vi "Get Matrix - file.vi"(7 "is string?":bool, 8 "error in (no error)":errorcluster, 10 "variable name":string, 11 "GOLPI ref. in":T1={"pipe handle"={"lv_proc.dll file path"=path "", "process instance handle"=[], "debug mode"=FALSE, "debug data"=[]}, "fast read timeout [ms]"=500, "fast read settle time [ms]"=10, "fast read to multiple [ms]"=1, "max elements per input line"=100, "slow read timeout [ms]"=5000, "stdin double format specifier"="%_16e", "max elements per stdout output column"=100, "console mode bitstream"=FALSE, "bitstream first read timeout [ms]"=1000, "bitstream read timeout [ms]"=50, "struct transfer possible"=FALSE, "matlab mode"=FALSE}) -> (0 "error out":errorcluster, 1 "cmplx double array":cdb[][](array[numeric]), 2 "double array":dbl[][](array[numeric]), 3 "GOLPI ref. out":T1={"pipe handle"={"lv_proc.dll file path"=path "", "process instance handle"=[], "debug mode"=FALSE, "debug data"=[]}, "fast read timeout [ms]"=500, "fast read settle time [ms]"=10, "fast read to multiple [ms]"=1, "max elements per input line"=100, "slow read timeout [ms]"=5000, "stdin double format specifier"="%_16e", "max elements per stdout output column"=100, "console mode bitstream"=FALSE, "bitstream first read timeout [ms]"=1000, "bitstream read timeout [ms]"=50, "struct transfer possible"=FALSE, "matlab mode"=FALSE}, 5 "string array":string[](array[string]))   [LabVIEW 2020, in "GOLPI library.lvlib"]
doc: "Saves GNU Octave variable into temporary file and loads it into LabVIEW. The variable is at the output terminal according to type of variable. Supported are reals (doubles), complex and strings. One has to select whether the variable is string."
uses:
  GOLPI library.lvlib
  GOLPI reference Type Def.ctl
  Pipe Handle.ctl
  Custom Error Codes Enum Type Def.vi
  LV Process library.lvlib
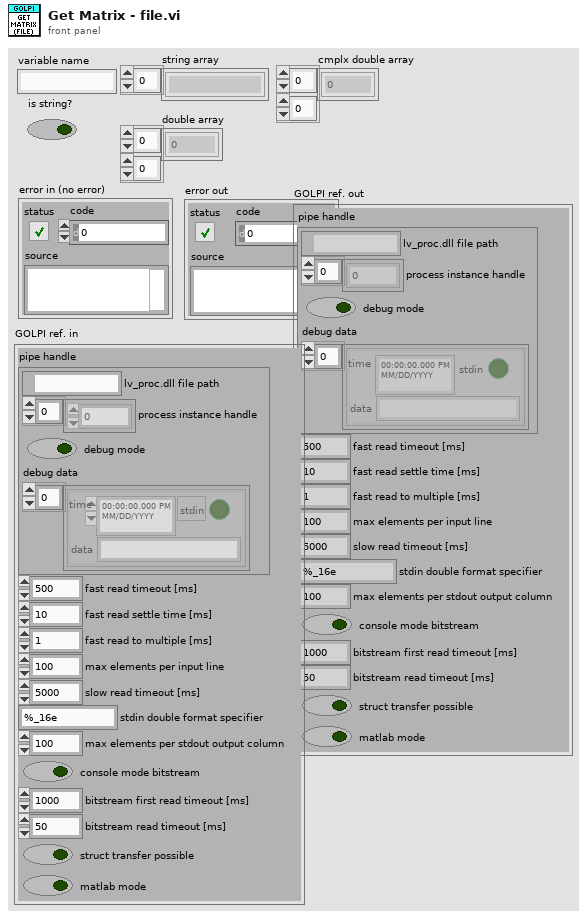
[diagram p1: front panel]
types:
  T1 = typedef "GOLPI library.lvlib/GOLPI reference Type Def.ctl" = cluster{"pipe handle":T2, "fast read timeout [ms]":u32, "fast read settle time [ms]":u32, "fast read to multiple [ms]":u32, "max elements per input line":u32, "slow read timeout [ms]":u32, "stdin double format specifier":string, "max elements per stdout output column":u32, "console mode bitstream":bool, "bitstream first read timeout [ms]":u32, "bitstream read timeout [ms]":u32, "struct transfer possible":bool, "matlab mode":bool}
  T2 = typedef "LV Process library.lvlib/Pipe Handle.ctl" = cluster{"lv_proc.dll file path":path, "process instance handle":u32[], "debug mode":bool, "debug data":cluster{"time":timestamp, "stdin":bool, "data":string}[]}
  T3 = typedef "GOLPI library.lvlib/Custom Error Codes Enum Type Def.vi" = enum16{"no error", "00 working directory PAR1 missing", "01 octave binary PAR1 missing", "02 octave report error PAR1", "03 empty output last cmd PAR1", "04 missing temporary file PAR1", "05 pwd PAR 1 not exist", "06 oct package not installed", "07 octave default binary missing", "10 var PAR1 not string, vect", "11 var PAR1 not num, scal, ~compl", "12 var PAR1 not num, scal, compl", "13 var PAR1 not num, vect, ~compl", "14 var PAR1 not num, vect, compl", "15 var PAR1 not num, mat, ~compl", "16 var PAR1 not num, mat, ~compl", "30 read timeout", "60 bitstream transport failed", "61 bitstream decode error PAR1", "62 bitstream cannot be set", "70 struct transfer not possible", "80 struct: cluster elem. PAR1 not implem.", "81 struct: structure field PAR1 not implem.", "82 struct: size mismatch of PAR1", "83 struct: type mismatch of PAR1", "98 internal error", "99 not finished", "90 Not supported in Matlab mode", "91 Matlab variable transfer error", "92 Matlab Script Error"}
  T4 = enum16{"open", "replace", "create", "open or create", "replace or create", "replace or create with confirmation"}
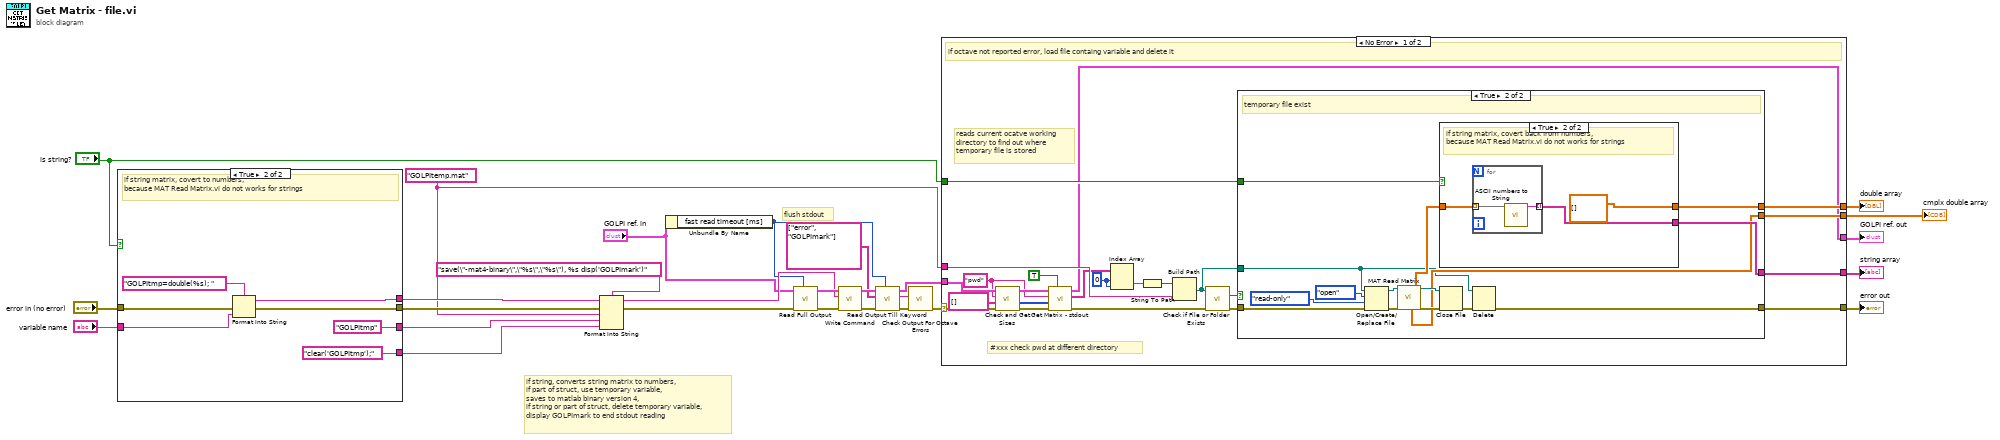
[diagram p0: block diagram]
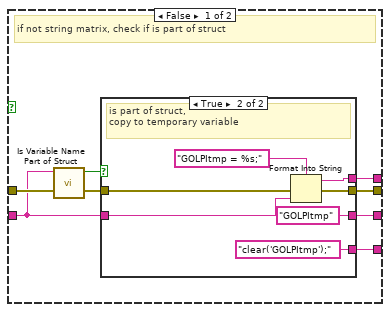
[diagram p2: hidden frame]
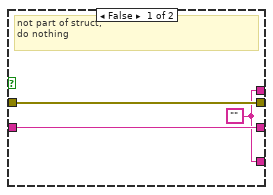
[diagram p3: hidden frame]
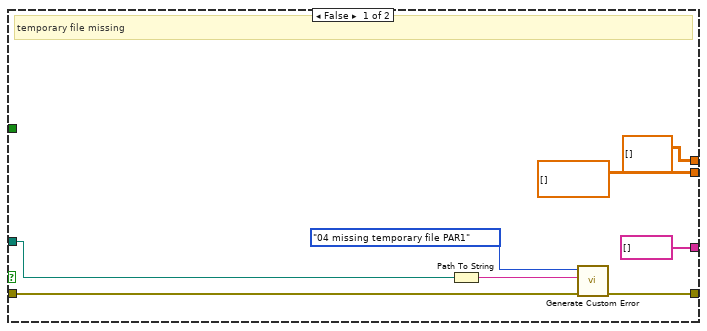
[diagram p4: hidden frame]
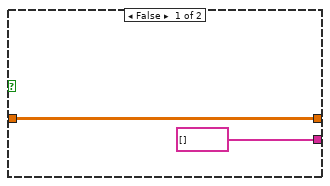
[diagram p5: hidden frame]
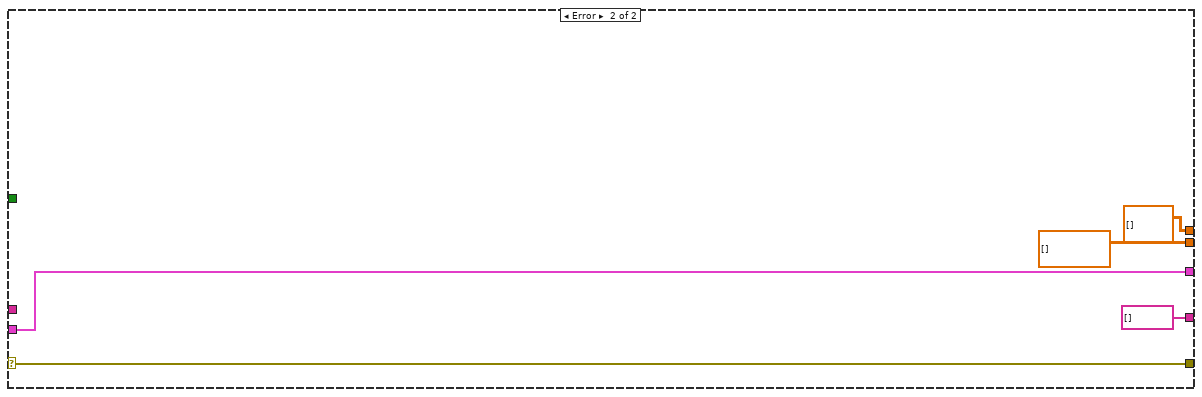
[diagram p6: hidden frame]
diagram:
  w7 = "GOLPItemp.mat" ("name or relative path")
  # "if string, converts string matrix to numbers,\nif part of struct, use temporary variable,\nsaves to matlab binary version 4,\nif string or part of struct, delete temporary variable,\ndisplay GOLPImark to end stdout reading"
  # "flush stdout"
  n1 = case shown="True" "is string?" {
    tunnel: [w33 w50] -> w14
    tunnel: [w30 "GOLPItmp" ("format string")] -> w15
    tunnel: "variable name" -> [w29 w48]
    tunnel: [w32 w46] -> w13
    tunnel: "error in (no error)" -> [w31 w47]
    tunnel: [w28 "clear('GOLPItmp');" ("format string")] -> w1
    frame False {
      # "if not string matrix, check if is part of struct"
      n2 = call "Is Variable Name Part of Struct.vi"("variable name"=w29) -> ("Is part of struct?"=w34:bool)  [unwired: 10 in]
      n3 = case shown="True" w34 {
        tunnel: [w35 w38] -> w33
        tunnel: [w37 w39] -> w32
        tunnel: w31 -> [w37 w40]
        tunnel: [w36 "GOLPItmp" ("f")] -> w30
        tunnel: w29 -> [w36 w41]
        tunnel: [w35 "clear('GOLPItmp');" ("format string")] -> w28
        frame False {
          w35 = ""
          # "not part of struct,\ndo nothing"
        }
        frame True {
          # "is part of struct,\ncopy to temporary variable"
          n4 = Format Into String(format string="GOLPItmp = %s;" ("f"), error in=w40, w41) -> (resulting string=w38:string, error out=w39:errorcluster)  [unwired: 1 in]
        }
      }
    }
    frame True {
      # "if string matrix, covert to numbers,\nbecause MAT Read Matrix.vi do not works for strings"
      n5 = Format Into String(format string="GOLPItmp=double(%s); ", error in=w47, w48) -> (resulting string=w50:string, error out=w46:errorcluster)  [unwired: 1 in]
    }
  }
  n6 = Format Into String(format string="save(\"-mat4-binary\",\"%s\",\"%s\"), %s disp('GOLPImark')", initial string=w14, error in=w13, w7, w15, w1) -> (resulting string=w18:string, error out=w24:errorcluster)
  n7 = Unbundle By Name("GOLPI ref. in") -> ("fast read timeout [ms]"=w4:u32)
  n8 = call "Read Full Output.vi"("timeout [ms]"=w4, "error in"=w24, "GOLPI ref. in"="GOLPI ref. in") -> ("error out"=w25:errorcluster, "GOLPI ref. out"=w26:T1)  [unwired: 5 in, 2 out]
  n9 = call "Write Command.vi"("error in"=w25, "command"=w18, "GOLPI ref. in"=w26) -> ("error out"=w23:errorcluster, "GOLPI ref. out"=w20:T1)  [unwired: 7 in]
  n10 = call "Read Output Till Keyword.vi"("timeout [ms]"=w4, "error in"=w23, "keywords"=string[] ["error", "GOLPImark"], "GOLPI ref. in"=w20) -> ("error out"=w22:errorcluster, "read buffer"=w21:string, "GOLPI ref. out"=w6:T1)  [unwired: 4 in, 1 out]
  n11 = call "Check Output For Octave Errors.vi"("error in"=w22, "read buffer"=w21) -> ("error out"=w17:errorcluster)  [unwired: 9 in]
  n12 = case shown="No Error" w17 {
    selector: w17 -> [w60 w109]
    tunnel: [w74 w109] -> w27
    tunnel: [w72 string[] []] -> w10
    tunnel: "is string?" -> [w73 _]
    tunnel: [w71 dbl[][] [] ("double array")] -> w9
    tunnel: [w70 cdb[][] [] ("CDB")] -> w8
    tunnel: w7 -> [w68 _]
    tunnel: w6 -> [w61 w105]
    tunnel: [w59 w105] -> w5
    frame No Error {
      w56 = 0 ("index (row)")
      w54 = "pwd" ("variable name")
      # "#xxx check pwd at different directory"
      # "reads current ocatve working\ndirectory to find out where\ntemporary file is stored"
      # "if octave not reported error, load file containg variable and delete it"
      n13 = call "Check and Get Sizes.vi"("error in (no error)"=w60, "test commands"=string[] [], "variable name"=w54, "GOLPI ref. in"=w61) -> ("error out"=w63:errorcluster, "octave sizes"=w53:i32[], "GOLPI ref. out"=w64:T1)  [unwired: 4 in, 1 out]
      n14 = call "Get Matrix - stdout.vi"("is string?"=TRUE ("is string"), "error in (no error)"=w63, "octave sizes"=w53, "variable name"=w54, "GOLPI ref. in"=w64) -> ("error out"=w58:errorcluster, "array"=w57:string[][], "GOLPI ref. out"=w59:T1)  [unwired: 4 in]
      n15 = Index Array(array=w57, index (row)=w56, index (col)=w56) -> (element=w55:string)
      n16 = String To Path(string=w55) -> (path=w69:path)
      n17 = Build Path(base path=w69, name or relative path=w68) -> (appended path=w66:path)
      n18 = call <vilib>:"Check if File or Folder Exists.vi"("error in (no error)"=w58, "path"=w66) -> ("error out"=w67:errorcluster, "file or folder exists?"=w65:bool)  [unwired: 7 in, 1 out]
      n19 = case shown="True" w65 {
        tunnel: [w81 w90] -> w74
        tunnel: w73 -> [_ w89]
        tunnel: [string[] [] w87] -> w72
        tunnel: [dbl[][] [] ("double array") w86] -> w71
        tunnel: [cdb[][] [] ("CDB") w85] -> w70
        tunnel: w67 -> [w82 w84]
        tunnel: w66 -> [w76 w83]
        frame False {
          # "temporary file missing"
          n20 = Path To String(path=w76) -> (string=w75:string)
          n21 = call "Generate Custom Error.vi"("error in"=w82, "PAR1"=w75, "GOLPI error"=Custom_Error_Codes_Enum_Type_Def.vi."04 missing temporary file PAR1" ("Enum")) -> ("error out"=w81:errorcluster)  [unwired: 8 in]
        }
        frame True {
          # "temporary file exist"
          n22 = Open/Create/Replace File(file path (use dialog)=w83, error in=w84, operation (0:open)=T4."open", access (0:read/write)=enum16{"read/write", "read-only", "write-only"}."read-only") -> (refnum out=w94:refnum<file>, error out=w96:errorcluster)  [unwired: 2 in, 1 out]
          n23 = call "MAT Read Matrix.vi"("Ref Num"=w94, "Error In"=w96) -> ("CDB"=w85:cdb[][], "DBL"=w88:dbl[][], "Dup Ref Num"=w95:refnum<file>, "error out"=w97:errorcluster)  [unwired: 5 in, 9 out]
          n24 = case shown="True" w89 {
            tunnel: w88 -> [w98 w102]
            tunnel: [string[] [] w101] -> w87
            tunnel: [w98 dbl[][] [] ("double array")] -> w86
            frame False {
            }
            frame True {
              # "if string matrix, covert back from numbers,\nbecause MAT Read Matrix.vi do not works for strings"
              n25 = for {
                tunnel: [w103] -> w101 mode=indexing
                tunnel: w102 -> [w104] mode=indexing
                n26 = call "ASCII numbers to String.vi"("ascii numbers"=w104) -> ("string"=w103:string)  [unwired: 10 in]
              }
            }
          }
          n27 = Close File(refnum=w95, error in=w97) -> (error out=w91:errorcluster)  [unwired: 1 out]
          n28 = Delete(path (use dialog)=w83, error in=w91) -> (error out=w90:errorcluster)  [unwired: 3 in, 2 out]
        }
      }
    }
    frame Error {
    }
  }
  "error out" <- w27
  "string array" <- w10
  "double array" <- w9
  "cmplx double array" <- w8
  "GOLPI ref. out" <- w5
